vi "Initialize Attributes.vi"(8 "error in (no error)":errorcluster, 10 "Attribute Data":variant, 11 "CS++DSCTrendViewer in":refnum<class "CS++DSCTrendViewer.lvclass">) -> (0 "error out":errorcluster, 2 "Found?":bool, 3 "CS++DSCTrendViewer out":refnum<class "CS++DSCTrendViewer.lvclass">)   [LabVIEW 2013, in "CS++DSCTrendViewer.lvlib" / "CS++DSCTrendViewer.lvclass"]
doc: "Initialize object attribute.\n\nUnique resources should be allocated elsewhere!"
uses:
  CS++DSCTrendViewer.lvclass
  CS++GUIActor/CS++GUIActor.lvclass
  CS++DSCTrendViewer.lvclass/CS++DSCTrendViewer.ctl
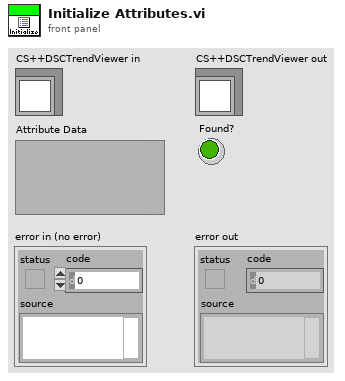
[diagram p1: front panel]
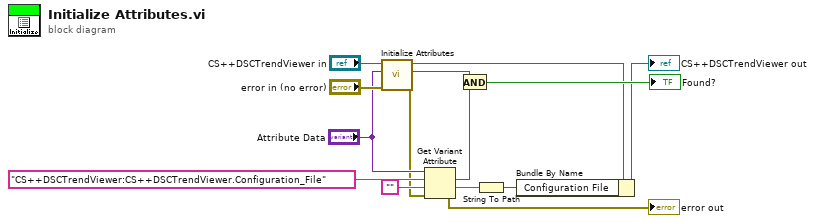
[diagram p0: block diagram]
diagram:
  n1 = call-parent "Initialize Attributes.vi"("error in (no error)"="error in (no error)", "Attribute Data"="Attribute Data", "CS++BaseActor in"="CS++DSCTrendViewer in") -> ("error out"=w9:errorcluster, "Found?"=w6:bool, "CS++BaseActor out"=w4:refnum<class "CS++DSCTrendViewer.lvclass">)  [unwired: 6 in]
  n2 = Get Variant Attribute(Variant="Attribute Data", name="CS++DSCTrendViewer:CS++DSCTrendViewer.Configuration_File", default value (empty Variant)="", error in=w9) -> (found=w7:bool, value=w2:string, error out=→"error out":errorcluster)  [unwired: 1 out]
  n3 = And(x=w6, y=w7) -> (x .and. y?=→"Found?":bool)
  n4 = String To Path(string=w2) -> (path=w1:path)
  n5 = Bundle By Name(cluster=w4, "Configuration File"=w1) -> (→"CS++DSCTrendViewer out":refnum<class "CS++DSCTrendViewer.lvclass">)
